vi "Wait.vi"(1 "milliseconds to wait":u32, 5 "error in (no error)":errorcluster) -> (19 "error out":errorcluster)   [LabVIEW 2017]
doc: "Waits the given number of milliseconds."
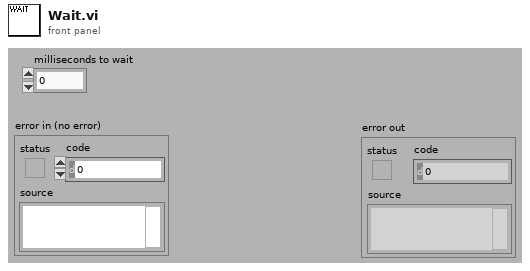
[diagram p1: front panel]
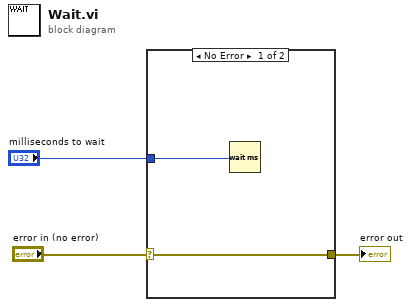
[diagram p0: block diagram]
diagram:
  n1 = case shown="No Error" "error in (no error)" {
    selector: "error in (no error)" -> [w5 w6]
    tunnel: [w5 w6] -> w2
    tunnel: "milliseconds to wait" -> [w4 _]
    frame No Error {
      n2 = Wait (ms)(milliseconds to wait=w4) -> ()  [unwired: 1 out]
    }
    frame Error {
    }
  }
  "error out" <- w2
